vi "create tdms file.vi"   [LabVIEW 2020]
types:
  T1 = enum16{"open", "open or create", "create or replace", "create", "open (read-only)"}
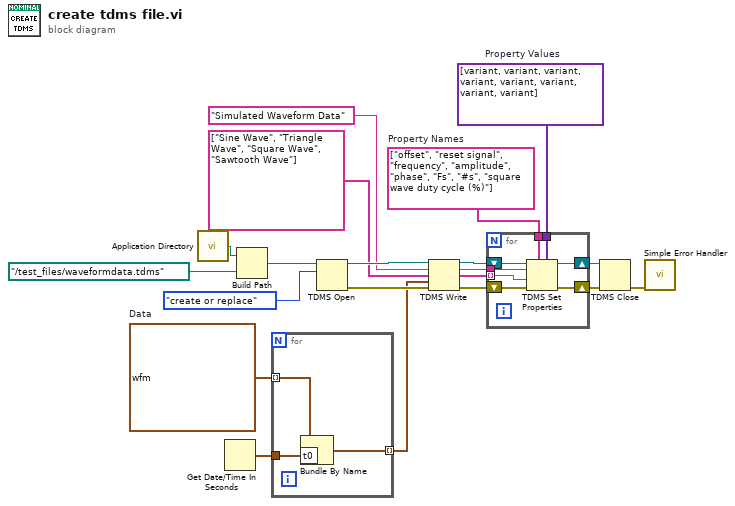
[diagram p0: block diagram]
diagram:
  w5 = variant[] [variant(dbl 0.0), variant(bool FALSE), variant(dbl 10.0), variant(dbl 1.0), variant(dbl 0.0), variant(dbl 1000.0), variant(dbl 1000.0), variant(dbl 50.0)]  # Property Values
  w4 = waveform(dbl)[] [{"t0"=timestamp(3829451887.3083134 s since 1904-01-01), "dt"=0.001, "Y"=array[1000 elements]}, {"t0"=timestamp(3829451887.3083134 s since 1904-01-01), "dt"=0.001, "Y"=array[1000 elements]}, {"t0"=timestamp(3829451887.3083134 s since 1904-01-01), "dt"=0.001, "Y"=array[1000 elements]}, {"t0"=timestamp(3829451887.3083134 s since 1904-01-01), "dt"=0.001, "Y"=array[1000 elements]}]  # Data
  w6 = string[] ["offset", "reset signal", "frequency", "amplitude", "phase", "Fs", "#s", "square wave duty cycle (%)"]  # Property Names
  n1 = call <vilib>:"Application Directory.vi"() -> ("Application Directory"=w16:path)
  n2 = Get Date/Time In Seconds() -> (seconds since 1Jan1904=w3:timestamp)
  n3 = Build Path(base path=w16, name or relative path=path "../test_files/waveformdata.tdms") -> (appended path=w14:path)
  n4 = for {
    tunnel: w4 -> [w23] mode=indexing
    tunnel: w3 -> [w22]
    tunnel: [w21] -> w2 mode=indexing
    n5 = Bundle By Name(cluster=w23, "t0"=w22) -> (w21:waveform(dbl))
  }
  n6 = TDMS Open(10:T1."create or replace" ("operation (0:open)"), 11:w14) -> (0:w19:errorcluster, 3:w20:refnum<k34>)  [unwired: 5 in]
  n7 = TDMS Write(0:w20, 5:"Simulated Waveform Data" ("group name in (Untitled)"), 7:string[] ["Sine Wave", "Triangle Wave", "Square Wave", "Sawtooth Wave"] ("Channel Names"), 9:w2, 11:w19) -> (4:w12:refnum<k34>, 6:w8:string, 8:w7:string[], 15:w9:errorcluster)  [unwired: 1 in]
  n8 = for {
    tunnel: w6 -> [w31]
    tunnel: w5 -> [w30]
    shift-right: [w28] -> w11
    shift-left: w12 -> [w29]
    shift-right: [w27] -> w10
    shift-left: w9 -> [w26]
    tunnel: w8 -> [w25]
    tunnel: w7 -> [w24] mode=indexing
    n9 = TDMS Set Properties(5:w30, 7:w31, 8:w26, 9:w24, 10:w25, 11:w29) -> (0:w27:errorcluster, 3:w28:refnum<k34>)  [unwired: 2 out]
  }
  n10 = TDMS Close(8:w10, 11:w11) -> (0:w1:errorcluster)  [unwired: 1 out]
  n11 = call <vilib>:"Simple Error Handler.vi"("error in (no error)"=w1) -> ()  [unwired: 4 in, 5 out]
